vi "Clamp AET Max_Vertical.vi"(0 "Image":T6, 1 "Rectangle":T8 {"Rotation" format="%.2f"; "Left" scale=0.0..1024.0; "Right" scale=0.0..1024.0}, 4 "Coordinate System":T7 {"Measurement System"."Axis Reference" items=["Direct", "Indirect"]; "Measurement System"."Angle (deg)" format="%.2f"; "Measurement System"."Origin"."Y" format="%.2f"; "Measurement System"."Origin"."X" format="%.2f"; "Reference System"."Axis Reference" items=["Direct", "Indirect"]; "Reference System"."Angle (deg)" format="%.2f"; "Reference System"."Origin"."Y" format="%.2f"; "Reference System"."Origin"."X" format="%.2f"}, 5 "error in (no error)":errorcluster, 6 "Settings":T5={"Contrast"=40, "Filter width"=4, "Steepness"=2, "Subsampling Ratio"=5, "Show Search Area"=FALSE, "Show Search Lines"=FALSE, "Show Edges Found"=FALSE, "Show Result"=TRUE}, 7 "Edge Options":T3={"Edge Polarity"=0, "Kernel Size"=3, "Width"=3, "Minimum Edge Strength"=10.0, "Interpolation Type"=enum."Bilinear Fixed", "Data Processing Method"=enum."Average"} {"Edge Polarity" items=["All Edges", "Rising Edges", "Falling Edges"]; "Minimum Edge Strength" format="%.2f"; "Width" step=2; "Kernel Size" step=2}) -> (10 "Edge Coordinates":cluster{"X":sgl, "Y":sgl}[](array[cluster]) {"Y" format="%.2f"; "X" format="%.2f"}, 13 "Search Lines":T2[](array[typedef]) {"Edge Info"."Distance (Real-World)" format="%.2f"; "Edge Info"."Location (Real-World)"."Y" format="%.2g"; "Edge Info"."Location (Real-World)"."X" format="%.2f"; "Edge Info"."Noise" format="%.2f"; "Edge Info"."Location (Pixel)"."Y" format="%.2g"; "Edge Info"."Location (Pixel)"."X" format="%.2f"; "Edge Info"."Strength" format="%.2f"; "Edge Info"."Distance (Pixel)" format="%.2f"}, 14 "Image Out":T6, 15 "Distance":sgl format="%.2f", 16 "First Edges":T1[](array[typedef]) {"Distance (Real-World)" format="%.2f"; "Location (Real-World)"."Y" format="%.2g"; "Location (Real-World)"."X" format="%.2f"; "Noise" format="%.2f"; "Location (Pixel)"."Y" format="%.2g"; "Location (Pixel)"."X" format="%.2f"; "Strength" format="%.2f"; "Distance (Pixel)" format="%.2f"}, 17 "Last Edges":T1[](array[typedef]) {"Distance (Real-World)" format="%.2f"; "Location (Real-World)"."Y" format="%.2g"; "Location (Real-World)"."X" format="%.2f"; "Noise" format="%.2f"; "Location (Pixel)"."Y" format="%.2g"; "Location (Pixel)"."X" format="%.2f"; "Strength" format="%.2f"; "Distance (Pixel)" format="%.2f"}, 18 "Coordinate System (duplicate)":T7 {"Measurement System"."Axis Reference" items=["Direct", "Indirect"]; "Measurement System"."Angle (deg)" format="%.2f"; "Measurement System"."Origin"."Y" format="%.2f"; "Measurement System"."Origin"."X" format="%.2f"; "Reference System"."Axis Reference" items=["Direct", "Indirect"]; "Reference System"."Angle (deg)" format="%.2f"; "Reference System"."Origin"."Y" format="%.2f"; "Reference System"."Origin"."X" format="%.2f"}, 19 "error out":errorcluster)   [LabVIEW 2019, in "Algorithm.lvclass"]
doc: "Modified NI Vertical Max Clamp with Rake-3 which uses Advanced Edge Detection."
uses:
  FrameworkOverrides/Algorithm.lvclass
  <vilib>/vision/NI_Vision_Development_Module.lvlib
  <vilib>/vision/Image Controls.llb/IMAQ Image.ctl
  <vilib>/vision/Measure.llb/Edge Polarity.ctl
  <vilib>/vision/Measure.llb/Edge Options.ctl
  <vilib>/vision/Measure.llb/Edge New.ctl
  <vilib>/vision/Measure.llb/Search Line.ctl
panel:
  out "Elapsed time (ms)":u32
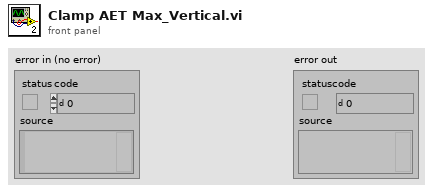
[diagram p1: front panel]
types:
  T1 = typedef "Edge New.ctl" = cluster{"Location (Pixel)":cluster{"X":sgl, "Y":sgl}, "Location (Real-World)":cluster{"X":sgl, "Y":sgl}, "Distance (Pixel)":dbl, "Distance (Real-World)":dbl, "Strength":dbl, "Noise":dbl, "Rising?":bool}
  T2 = typedef "Search Line.ctl" = cluster{"Start Point":cluster{"X":sgl, "Y":sgl}, "End Point":cluster{"X":sgl, "Y":sgl}, "Edge Info":T1[], "Edge Map":dbl[], "Calibration Valid":bool}
  T3 = typedef "Edge Options.ctl" = cluster{"Edge Polarity":T4, "Kernel Size":u32, "Width":u32, "Minimum Edge Strength":sgl, "Interpolation Type":enum32{"Zero Order", "Bilinear", "Quadratic", "Cubic", "Bilinear Fixed"}, "Data Processing Method":enum32{"Average", "Median"}}
  T4 = typedef "Edge Polarity.ctl" = u32
  T5 = cluster{"Contrast":i32, "Filter width":i32, "Steepness":i32, "Subsampling Ratio":u32, "Show Search Area":bool, "Show Search Lines":bool, "Show Edges Found":bool, "Show Result":bool}
  T6 = typedef "IMAQ Image.ctl" = refnum<image>
  T7 = typedef "IMAQ Coordinate System" = cluster{"Reference System":cluster{"Origin":cluster{"X":sgl, "Y":sgl}, "Angle (deg)":sgl, "Axis Reference":u32}, "Measurement System":cluster{"Origin":cluster{"X":sgl, "Y":sgl}, "Angle (deg)":sgl, "Axis Reference":u32}}
  T8 = typedef "IMAQ Rectangle" = cluster{"Left":i32, "Top":i32, "Right":i32, "Bottom":i32, "Rotation":dbl}
  T9 = enum16{"Get First Edge", "Get First + Last Edge", "Get All Edges", "Get Best Edge"}
  T10 = cluster{"Start Point":cluster{"X":sgl, "Y":sgl}, "End Point":cluster{"X":sgl, "Y":sgl}}
  T11 = typedef "ROI Descriptor" = cluster{"Global Rectangle":i32[], "Contours":cluster{"ID":enum32{"External", "Internal"}, "Type":u32, "Coordinates":i32[]}[]}
  T12 = cluster{cluster{"X":sgl, "Y":sgl}, cluster{"X":sgl, "Y":sgl}}[]
  T13 = cluster{"Show Search Area":bool, "Show Search Lines":bool, "Show Edges Found":bool, "Show Result":bool}
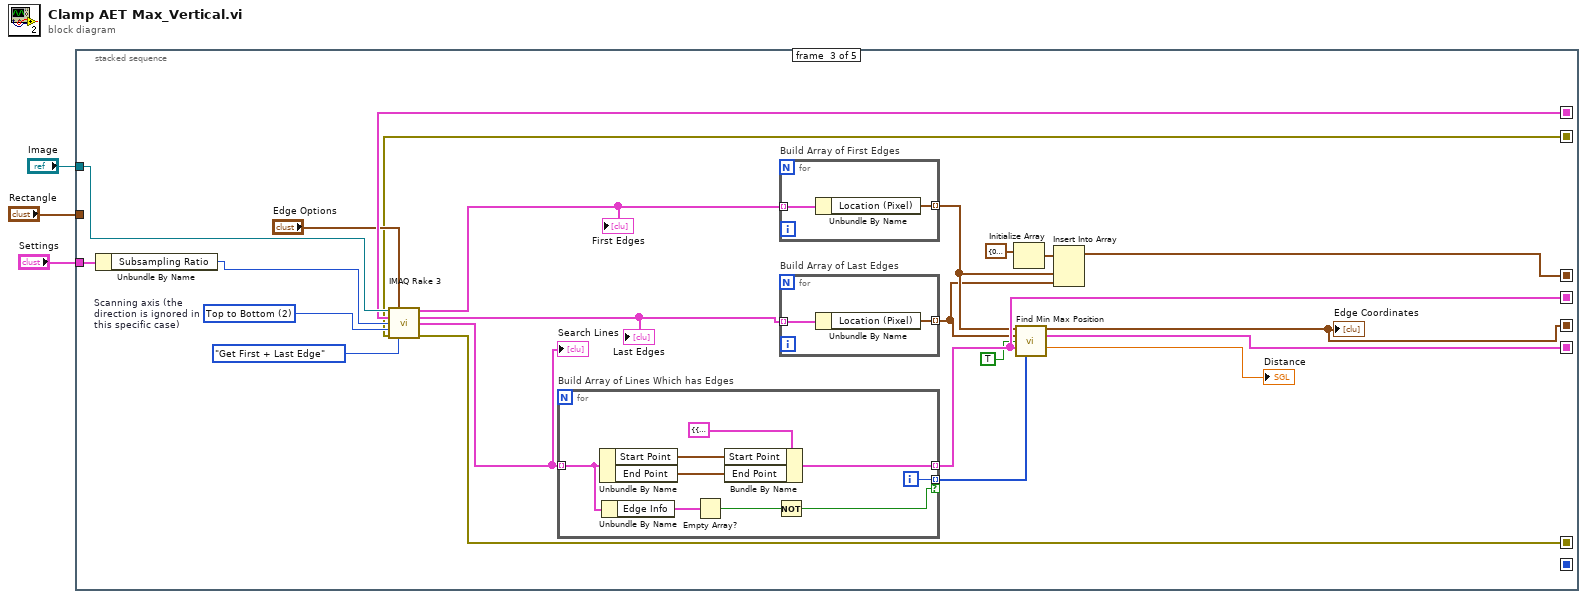
[diagram p0: block diagram]
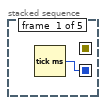
[diagram p2: hidden frame]
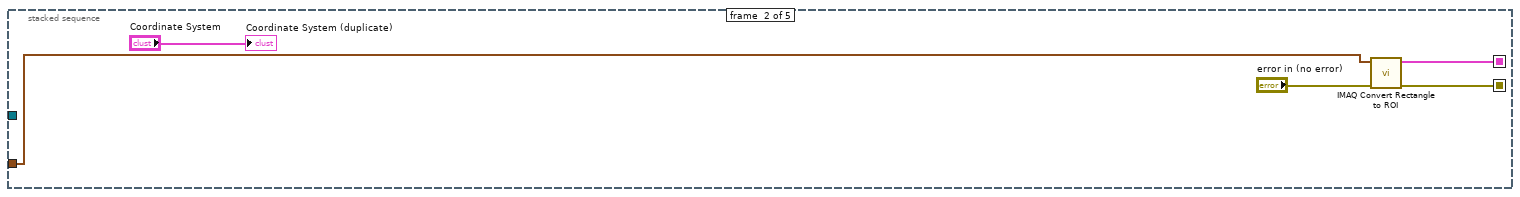
[diagram p3: hidden frame]
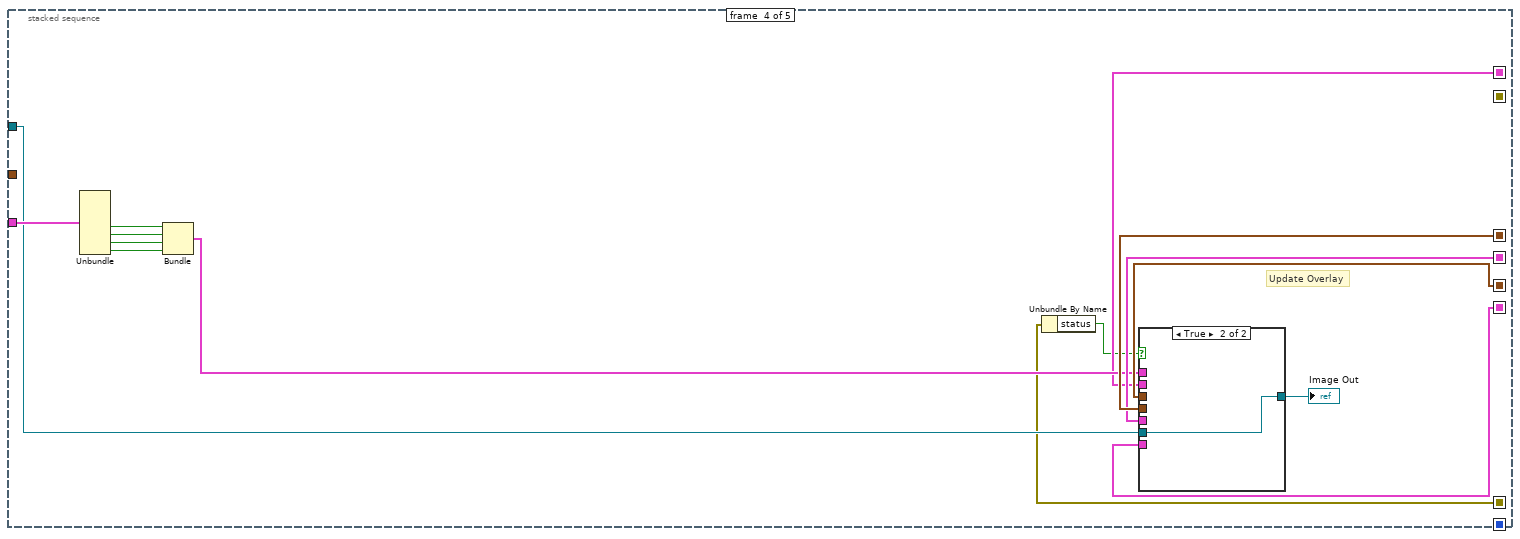
[diagram p4: hidden frame]
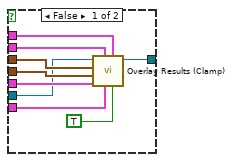
[diagram p5: hidden frame]
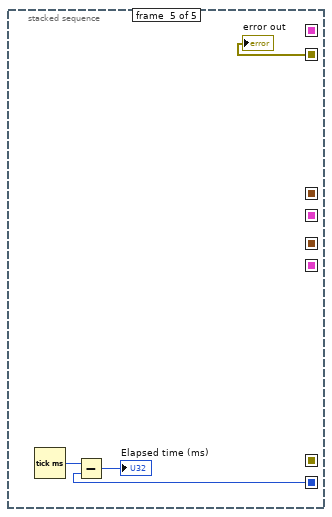
[diagram p6: hidden frame]
diagram:
  n1 = stacked-sequence {
    seq-local: [_ _ w21 _ _] -> [_ _ _ w60 _]
    seq-local: [w4 _ _ _ _] -> [_ _ _ _ w74]
    seq-local: [_ _ w10 _ _] -> [_ _ _ w59 _]
    seq-local: [_ _ w23 _ _] -> [_ _ _ w58 _]
    seq-local: [_ _ w22 _ _] -> [_ _ _ w52 _]
    seq-local: [_ w5 _ _ _] -> [_ _ w30 w50 _]
    seq-local: [_ w7 _ _ _] -> [_ _ w17 _ w71]
    seq-local: [_ _ w16 _ _] -> [_ _ _ w46 _]
    tunnel: "Image" -> [_ _ w31 w49 _]
    tunnel: "Rectangle" -> [_ w8 _ _ _]
    tunnel: "Settings" -> [_ _ w32 w57 _]
    frame #0 {
      n2 = Tick Count (ms)() -> (millisecond timer value=w4:u32)
    }
    frame #1 {
      n3 = call "IMAQ Convert Rectangle to ROI"("error in (no error)"="error in (no error)", "Rectangle"=w8) -> ("error out"=w7:errorcluster, "ROI Descriptor"=w5:T11)  [unwired: 7 out]
      "Coordinate System (duplicate)" <- "Coordinate System"
    }
    frame #2 {
      w28 = u32 2 items=["Left to Right", "Right to Left", "Top to Bottom", "Bottom to Top"]  # Scanning axis (the direction is ignored in this specific case)
      n4 = Unbundle By Name(w32) -> ("Subsampling Ratio"=w29:u32)
      n5 = call "IMAQ Rake 3"("Image"=w31, "Edge Options"="Edge Options", "ROI Descriptor"=w30, "Step Size"=w29, "Scan Direction"=w28, "error in (no error)"=w17, "Process"=T9."Get First + Last Edge") -> ("First Edges"=w26:T1[], "Last Edges"=w25:T1[], "Search Lines"=w24:T2[], "error out"=w16:errorcluster)  [unwired: 5 in]
      "Search Lines" <- w24
      "First Edges" <- w26
      "Last Edges" <- w25
      n6 = for "Build Array of Lines Which has Edges" {
        tunnel: w24 -> [w38] mode=indexing
        tunnel: [w39] -> w23 mode=indexing
        tunnel: [w35] -> w19 mode=indexing if=w34
        i -> [w35]
        n7 = Unbundle By Name(w38) -> ("Start Point"=w41:cluster{"X":sgl, "Y":sgl}, "End Point"=w40:cluster{"X":sgl, "Y":sgl})
        n8 = Unbundle By Name(w38) -> ("Edge Info"=w37:T1[])
        n9 = Empty Array?(array=w37) -> (empty?=w36:bool)
        n10 = Bundle By Name(cluster=T10 {"Start Point"={"X"=0.0, "Y"=0.0}, "End Point"={"X"=0.0, "Y"=0.0}} ("Cluster 2"), "Start Point"=w41, "End Point"=w40) -> (w39:T10)
        n11 = Not(x=w36) -> (.not. x?=w34:bool)
      }
      n12 = for "Build Array of First Edges" {
        tunnel: w26 -> [w45] mode=indexing
        tunnel: [w44] -> w12 mode=indexing
        n13 = Unbundle By Name(w45) -> ("Location (Pixel)"=w44:cluster{"X":sgl, "Y":sgl})
      }
      n14 = for "Build Array of Last Edges" {
        tunnel: w25 -> [w43] mode=indexing
        tunnel: [w42] -> w11 mode=indexing
        n15 = Unbundle By Name(w43) -> ("Location (Pixel)"=w42:cluster{"X":sgl, "Y":sgl})
      }
      n16 = Initialize Array(cluster{"X":sgl, "Y":sgl} {"X"=0.0, "Y"=0.0} ("Real World Coordinates")) -> (w13:cluster{"X":sgl, "Y":sgl}[])  [unwired: 1 in]
      n17 = call "Find Min Max Position.vi"("First Edges"=w12, "Last Edges"=w11, "Min / Max"=TRUE, "Search Lines"=w23, "Lines with Edges (first)"=w19) -> ("Points"=w21:cluster{"X":sgl, "Y":sgl}[], "Perpendicular Lines"=w22:T12, "Distance"=→"Distance":sgl)  [unwired: 7 in, 1 out]
      "Edge Coordinates" <- w21
      n18 = Insert Into Array(array=w13, new element #1=w12, new element #2=w11) -> (w10:cluster{"X":sgl, "Y":sgl}[])  [unwired: 1 in]
    }
    frame #3 {
      # "Update Overlay"
      n19 = Unbundle(w57) -> ("Show Search Area"=w56:bool, "Show Search Lines"=w55:bool, "Show Edges Found"=w54:bool, "Show Result"=w53:bool)  [unwired: 4 out]
      n20 = Bundle("Show Search Area"=w56, "Show Search Lines"=w55, "Show Edges Found"=w54, "Show Result"=w53) -> (w51:T13)  [unwired: 1 out]
      n21 = Unbundle By Name(w46) -> ("status"=w47:bool)
      n22 = case shown="True" w47 {
        tunnel: w60 -> [w69 _]
        tunnel: w59 -> [w68 _]
        tunnel: w58 -> [w67 _]
        tunnel: w52 -> [w66 _]
        tunnel: w51 -> [w64 _]
        tunnel: w50 -> [w63 _]
        tunnel: w49 -> [w62 w70]
        tunnel: [w61 w70] -> w48
        frame False {
          n23 = call <vilib>:"Overlay Results (Clamp).vi"("Min / Max"=TRUE, "Setup"=w64, "Perpendicular Lines"=w66, "ROI Descriptor"=w63, "Search Lines"=w67, "All Edges Found"=w68, "Measurement Edges"=w69, "Image In"=w62) -> ("Image Out"=w61:T6)  [unwired: 3 out]
        }
        frame True {
        }
      }
      "Image Out" <- w48
    }
    frame #4 {
      n24 = Tick Count (ms)() -> (millisecond timer value=w73:u32)
      n25 = Subtract(x=w73, y=w74) -> (x-y=→"Elapsed time (ms)":u32)
      "error out" <- w71
    }
  }
